vi "eval Command.vi"(8 "error in (no error)":errorcluster caption="Fehler (Eingang, kein Fehler)", 10 "Commandline":string, 11 "TestInterface.lvclass":refnum<class "TestInterface.lvclass">) -> (0 "error out":errorcluster caption="Fehler (Ausgang)", 1 "isQuerry":bool, 2 "timeout(ms)":i32, 3 "TestInterface.lvclass 2":refnum<class "TestInterface.lvclass">, 4 "wait":u32)   [LabVIEW 2013, in "TestInterface.lvclass"]
doc: "In diesem VI wird beurteilt, wie auf den aktuellen Befehl reagiert werden soll. Wenn der aktuelle Befehl auf einen der hinterlegten regulären Ausdrücke passt, wird ein angepasstes Verhalten ausgeführt."
uses:
  TestInterface.lvclass
  <vilib>/regexp/Match Regular Expression.xnode
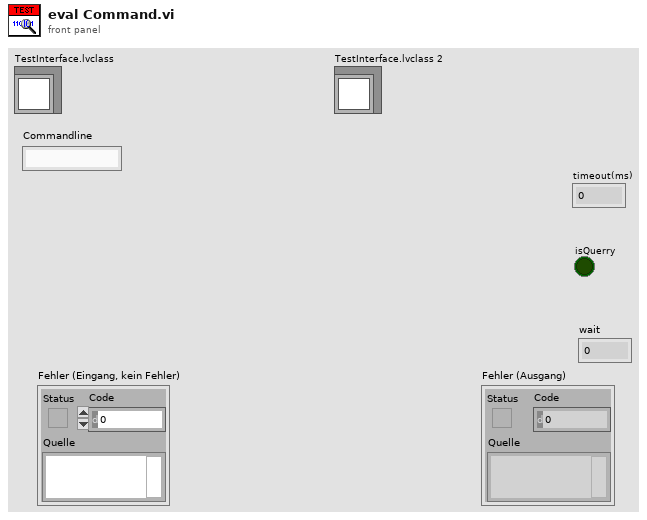
[diagram p1: front panel]
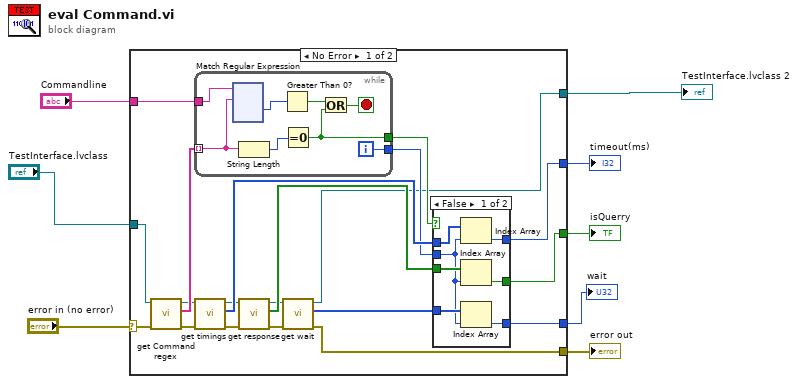
[diagram p0: block diagram]
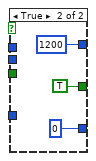
[diagram p2: hidden frame]
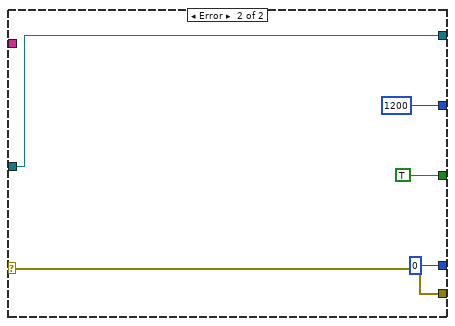
[diagram p3: hidden frame]
diagram:
  n1 = case shown="No Error" "error in (no error)" {
    selector: "error in (no error)" -> [w26 w165]
    tunnel: [w10 w165] -> w7
    tunnel: "Commandline" -> [w28 _]
    tunnel: "TestInterface.lvclass" -> [w27 w164]
    tunnel: [w9 w164] -> w1
    tunnel: [w20 TRUE ("Boolesch")] -> w5
    tunnel: [w19 1200 ("Numerisch")] -> w4
    tunnel: [w11 0 ("Numerisch")] -> w3
    frame No Error {
      n2 = call-dynamic "get Command regex.vi"("error in (no error)"=w26, "TestInterface (Eingang)"=w27) -> ("error out"=w17:errorcluster, "Command regex"=w25:string[], "TestInterface (Ausgang)"=w22:refnum<class "TestInterface.lvclass">)  [unwired: 7 in]
      n3 = while {
        tunnel: w28 -> [w41]
        tunnel: w25 -> [w40] mode=indexing
        tunnel: [w43] -> w23
        tunnel: [w42] -> w15
        i -> [w43]
        stop <- w45 stop-if-true
        n4 = xnode "Match Regular Expression"("input string"=w41, "regular expression"=w40) -> ("offset past match"=w39:i32)  [unwired: 4 in, 4 out]
        n5 = String Length(string=w40) -> (length=w46:i32)
        n6 = Greater Than 0?(x=w39) -> (x > 0?=w44:bool)
        n7 = Equal To 0?(x=w46) -> (x = 0?=w42:bool)
        n8 = Or(x=w44, y=w42) -> (x .or. y?=w45:bool)
      }
      n9 = call-dynamic "get timings.vi"("error in (no error)"=w17, "TestInterface (Eingang)"=w22) -> ("error out"=w16:errorcluster, "timings"=w24:i32[], "TestInterface (Ausgang)"=w18:refnum<class "TestInterface.lvclass">)  [unwired: 7 in]
      n10 = call-dynamic "get response.vi"("error in (no error)"=w16, "TestInterface (Eingang)"=w18) -> ("error out"=w14:errorcluster, "response?"=w21:bool[], "TestInterface (Ausgang)"=w13:refnum<class "TestInterface.lvclass">)  [unwired: 7 in]
      n11 = call-dynamic "get wait.vi"("error in (no error)"=w14, "TestInterface in"=w13) -> ("error out"=w10:errorcluster, "wait"=w12:u32[], "TestInterface out"=w9:refnum<class "TestInterface.lvclass">)  [unwired: 7 in]
      n12 = case shown="False" w15 {
        tunnel: w24 -> [w35 _]
        tunnel: w23 -> [w30 _]
        tunnel: w21 -> [w34 _]
        tunnel: [w33 TRUE ("Boolesch")] -> w20
        tunnel: [w32 1200 ("Numerisch")] -> w19
        tunnel: w12 -> [w31 _]
        tunnel: [w29 u32 0 ("Numerisch")] -> w11
        frame False {
          n13 = Index Array(array=w35, index=w30) -> (element=w32:i32)
          n14 = Index Array(array=w34, index=w30) -> (element=w33:bool)
          n15 = Index Array(array=w31, index=w30) -> (element=w29:u32)
        }
        frame True {
        }
      }
    }
    frame Error {
    }
  }
  "error out" <- w7
  "timeout(ms)" <- w4
  "isQuerry" <- w5
  "wait" <- w3
  "TestInterface.lvclass 2" <- w1
